vi "FTW-Ether-CreateEndpoint.vi"(5 "Endpoint Type":T2, 7 "Message Transport Scheme":T1, 11 "error in":errorcluster) -> (4 "FTW Endpoint":refnum<class "FTW-Endpoint.lvclass">, 15 "error out":errorcluster)   [LabVIEW 2012, in "FTW-Actor.lvlib" / "FTW-Ether.lvclass"]
uses:
  FTW-Ether.lvclass
  Endpoint/FTW-Endpoint.lvclass
  FTW-Ether-EndpointType.ctl
  FTW-Ether-MessageTransportScheme.ctl
  ZMQ/FTW-ZMQ-SocketType.ctl
  FTW-Ether-Instance.vi
  ZMQ/FTW-Endpoint-ZMQ.lvclass
panel:
  # "Inputs"
  # "Outputs"
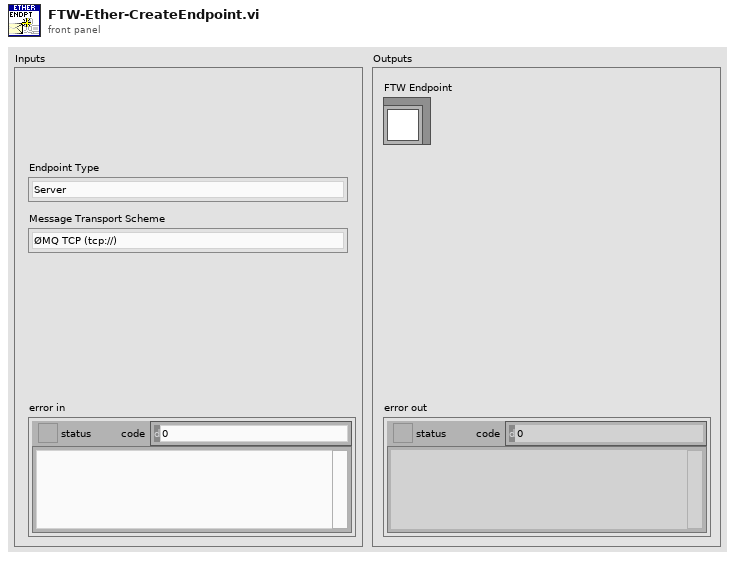
[diagram p1: front panel]
types:
  T1 = typedef "FTW-Actor.lvlib/FTW-Ether.lvclass/FTW-Ether-MessageTransportScheme.ctl" = enum16{"ØMQ TCP (tcp://)", "ØMQ In-Process (inproc://)", "LabVIEW Queues (lvq://)", "LabVIEW Network Streams (lvns://)"}
  T2 = typedef "FTW-Actor.lvlib/FTW-Ether.lvclass/FTW-Ether-EndpointType.ctl" = enum16{"Server", "Client", "Publisher", "Subscriber"}
  T3 = typedef "FTW-Endpoint-ZMQ.lvclass/FTW-ZMQ-SocketType.ctl" = enum32{"ZMQ_PAIR", "ZMQ_PUB", "ZMQ_SUB", "ZMQ_REQ", "ZMQ_REP", "ZMQ_DEALER", "ZMQ_ROUTER", "ZMQ_PULL", "ZMQ_PUSH", "ZMQ_XPUB", "ZMQ_XSUB", "ZMQ_STREAM"}
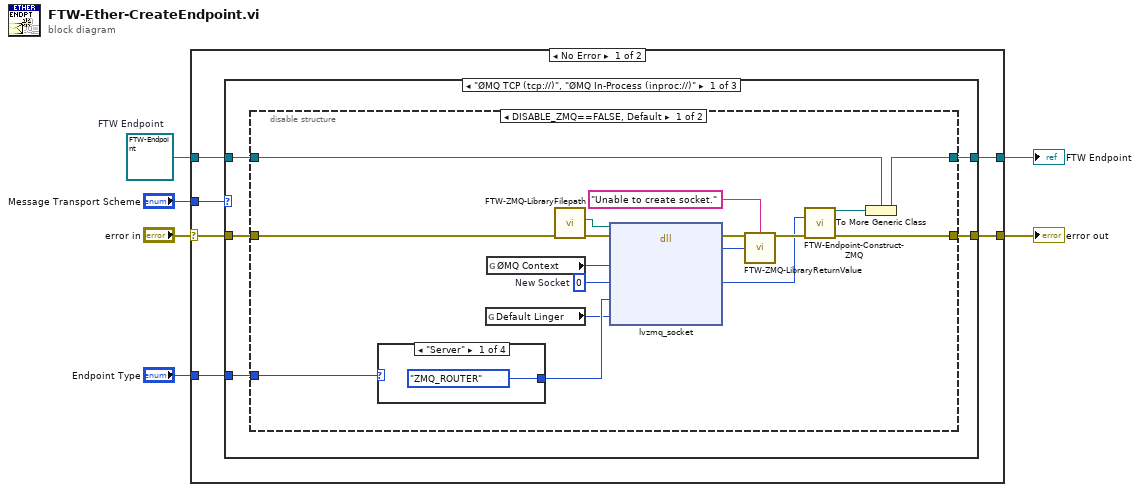
[diagram p0: block diagram]
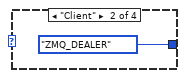
[diagram p2: hidden frame]
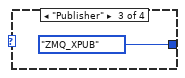
[diagram p3: hidden frame]
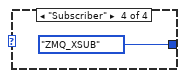
[diagram p4: hidden frame]
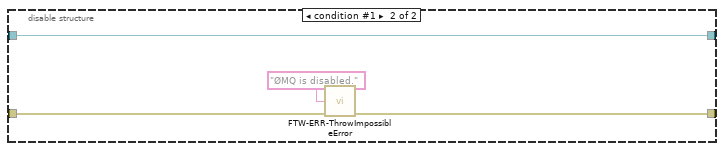
[diagram p5: hidden frame]
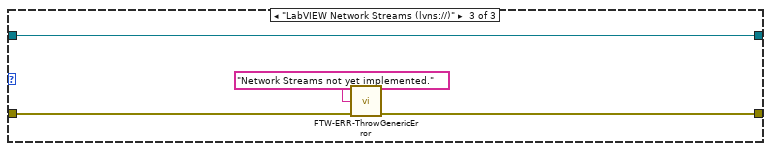
[diagram p7: hidden frame]
diagram:
  w1 = refnum<class "FTW-Endpoint.lvclass"> refnum  # FTW Endpoint
  n1 = case shown="No Error" "error in" {
    selector: "error in" -> [w9 w50]
    tunnel: [w12 w49] -> w6
    tunnel: [w11 w50] -> w5
    tunnel: "Message Transport Scheme" -> [w10 _]
    tunnel: "Endpoint Type" -> [w8 _]
    tunnel: w1 -> [w7 w49]
    frame No Error {
      n2 = case shown="\"ØMQ TCP (tcp://)\", \"ØMQ In-Process (inproc://)\"" w10 {
        tunnel: [w14 w43 w45] -> w12
        tunnel: [w17 w44 w46] -> w11
        tunnel: w9 -> [w16 w44 w47]
        tunnel: w8 -> [w15 _ _]
        tunnel: w7 -> [w13 w43 w45]
        frame "ØMQ TCP (tcp://)", "ØMQ In-Process (inproc://)" {
          n3 = disable-structure shown="DISABLE_ZMQ==FALSE, Default" {
            disable-tunnel: [w20 w39] -> w14
            disable-tunnel: [w34 w41] -> w17
            disable-tunnel: w16 -> [w32 w42]
            disable-tunnel: w15 -> [w33 _]
            disable-tunnel: w13 -> [w21 w39]
            frame condition #0 (active) {
              w28 = u64 0  # New Socket
              n4 = case shown="\"Server\"" w33 {
                tunnel: [FTW-ZMQ-SocketType."ZMQ_ROUTER" ("Socket Type") FTW-ZMQ-SocketType."ZMQ_DEALER" ("Socket Type") FTW-ZMQ-SocketType."ZMQ_XPUB" ("Socket Type") FTW-ZMQ-SocketType."ZMQ_XSUB" ("Socket Type")] -> w29
                frame "Server" {
                }
                frame "Client" {
                }
                frame "Publisher" {
                }
                frame "Subscriber" {
                }
              }
              n5 = global read "FTW-Ether-Instance.vi" "Default Linger"() -> (w18:i32)
              n6 = global read "FTW-Ether-Instance.vi" "ØMQ Context"() -> (w19:u64)
              n7 = call "FTW-ZMQ-LibraryFilepath.vi"("error in"=w32) -> ("error out"=w27:errorcluster, "FTW-ZMQ Library Filepath"=w23:path)  [unwired: 8 in, 1 out]
              n8 = dll-call lib="?" fn="lvzmq_socket"(path in=w23, error in=w27, "Context"=w19, "New Socket"=w28, "Socket Type"=w29, "Linger (msec)"=w18) -> (error out=w25:errorcluster, "Return Value"=w26:i32, "New Socket"=w30:u64)  [unwired: 4 in, 1 out]
              n9 = call "FTW-ZMQ-LibraryReturnValue.vi"("error in"=w25, "Error Message"="Unable to create socket.", "Return Value"=w26) -> ("error out"=w31:errorcluster)  [unwired: 12 in]
              n10 = call "FTW-Endpoint-Construct-ZMQ.vi"("Socket Pointer"=w30, "error in"=w31) -> ("FTW ØMQ Endpoint"=w22:refnum<class "FTW-Endpoint-ZMQ.lvclass">, "error out"=w34:errorcluster)  [unwired: 12 in]
              n11 = To More Generic Class(target class=w21, reference=w22) -> (generic class reference=w20:refnum<class "FTW-Endpoint.lvclass">)
            }
            frame condition #1 {
              n12 = call "FTW-ERR-ThrowImpossibleError.vi"("Reason this error should never happen"="ØMQ is disabled." ("Error Message"), "error in"=w42) -> ("error out"=w41:errorcluster)  [unwired: 13 in]
            }
          }
        }
        frame "LabVIEW Queues (lvq://)" {
        }
        frame "LabVIEW Network Streams (lvns://)" {
          n13 = call "FTW-ERR-ThrowGenericError.vi"("Error Message"="Network Streams not yet implemented.", "error in"=w47) -> ("error out"=w46:errorcluster)  [unwired: 13 in]
        }
      }
    }
    frame Error {
    }
  }
  "error out" <- w5
  "FTW Endpoint" <- w6
